vi "Create WavBuf.vi"(5 "Scale Offset":T2={"Slope"=1.0, "Intercept"=0.0} {"Intercept" format="%.6g"; "Slope" format="%.6g"}, 6 "Units":string, 7 "Name":string, 8 "Error":errorcluster, 9 "Task Timing":T1={"Buffer Size (S)"=7200.0, "rate (S/sec)"=2.0}, 11 "WavBuf":refnum<class "WavBuf.lvclass">) -> (0 "Error Out":errorcluster, 3 "WavBuf Out":refnum<class "WavBuf.lvclass">)   [LabVIEW 2020, in "WavBuf.lvclass"]
uses:
  WavBuf.lvclass
  TypeDefs_Utility/Cluster_Slope and Intercept.ctl
  TypeDefs_Utility/Cluster_Buffer and Rate.ctl
  Pointer/_Pointer.lvclass
  Universal Controls/Read Write Button.ctl
  Universal Controls/Waveform_Data.ctl
  WavBuf.lvclass/WavBuf.ctl
  error/Error Eater.vi
  <vilib>/Utility/LVClass/Get LV Class Name.vi
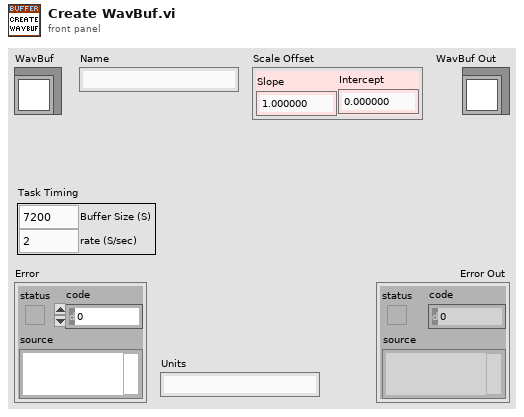
[diagram p1: front panel]
types:
  T1 = typedef "Cluster_Buffer and Rate.ctl" = cluster{"Buffer Size (S)":dbl, "rate (S/sec)":dbl}
  T2 = typedef "Cluster_Slope and Intercept.ctl" = cluster{"Slope":dbl, "Intercept":dbl}
  T3 = typedef "Waveform_Data.ctl" = waveform(dbl)
  T4 = typedef "Read Write Button.ctl" = bool
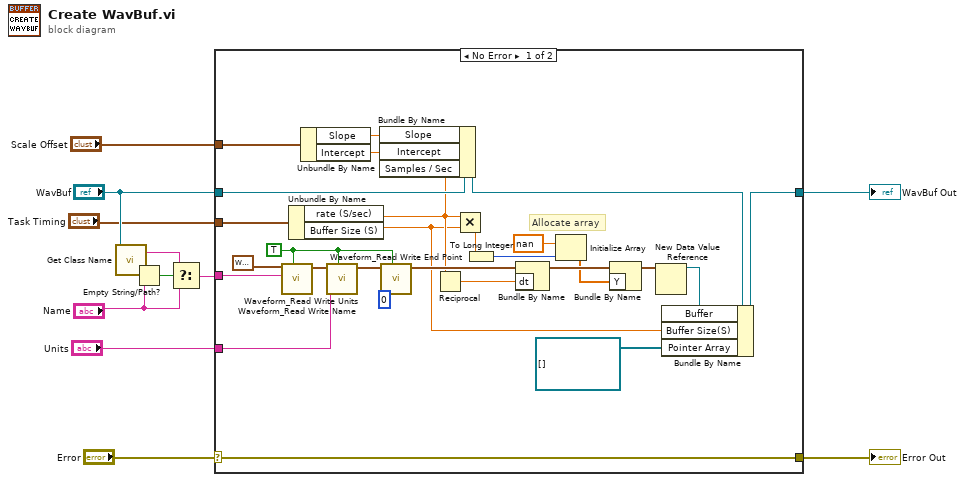
[diagram p0: block diagram]
diagram:
  n1 = call "Get Class Name.vi"("lvclass"="WavBuf") -> ("Child Name"=w7:string)  [unwired: 3 in, 1 out]
  n2 = Empty String/Path?(string/path="Name") -> (empty?=w8:bool)
  n3 = Select(t=w7, s=w8, f="Name") -> (s? t:f=w5:string)
  n4 = case shown="No Error" "Error" {
    selector: "Error" -> [w38 w40]
    tunnel: [w38 w40] -> w10
    tunnel: [w37 w39] -> w4
    tunnel: "WavBuf" -> [w29 w39]
    tunnel: w5 -> [w34 _]
    tunnel: "Units" -> [w19 _]
    tunnel: "Task Timing" -> [w17 _]
    tunnel: "Scale Offset" -> [w14 _]
    frame No Error {
      w18 = T4 TRUE ("Read(f)\nWrite(t)")
      # "Allocate array"
      n5 = call "Waveform_Read Write Name.vi"("Read(f)\nWrite(t)"=w18, "Name"=w34, "Raw Data Waveform"=T3 {"t0"=timestamp(0 s since 1904-01-01), "dt"=1.0, "Y"=[]}) -> ("Raw Data Waveform Out"=w21:T3)  [unwired: 7 in, 1 out]
      n6 = Unbundle By Name(w17) -> ("rate (S/sec)"=w16:dbl, "Buffer Size (S)"=w15:dbl)
      n7 = Unbundle By Name(w14) -> ("Slope"=w13:dbl, "Intercept"=w12:dbl)
      n8 = call "Waveform_Read Write Units.vi"("Read(f)\nWrite(t)"=w18, "Name"=w19, "Raw Data Waveform"=w21) -> ("Raw Data Waveform Out"=w20:T3)  [unwired: 7 in, 1 out]
      n9 = Bundle By Name(cluster=w29, "Slope"=w13, "Intercept"=w12, "Samples / Sec"=w16) -> (w28:refnum<class "WavBuf.lvclass">)
      n10 = call "Waveform_Read Write End Point.vi"("Read(f)\nWrite(t)"=w18, "End Point"=0, "Raw Data Waveform"=w20) -> ("Raw Data Waveform Out"=w27:T3)  [unwired: 7 in, 1 out]
      n11 = Reciprocal(x=w16) -> (1/x=w30:dbl)
      n12 = Multiply(x=w16, y=w15) -> (x*y=w22:dbl)
      n13 = To Long Integer(number=w22) -> (32bit integer=w23:i32)
      n14 = Bundle By Name(cluster=w27, "dt"=w30) -> (w31:T3)
      n15 = Initialize Array(nan ("Buffer Size(S)"), w23) -> (w24:dbl[])
      n16 = Bundle By Name(cluster=w31, "Y"=w24) -> (w33:T3)
      n17 = New Data Value Reference(data value=w33) -> (data value reference=w36:refnum<data-value>)  [unwired: 1 in, 1 out]
      n18 = Bundle By Name(cluster=w28, "Buffer"=w36, "Buffer Size(S)"=w15, "Pointer Array"=refnum<class "_Pointer.lvclass">[] []) -> (w37:refnum<class "WavBuf.lvclass">)
    }
    frame Error {
    }
  }
  "Error Out" <- w10
  "WavBuf Out" <- w4
